vi "Send Write CPU View.vi"(7 "Message Priority (Normal)":T2=enum."Normal", 8 "error in (no error)":errorcluster, 10 "CPU View":T1 {"fwidth:" format="%#_6p"; "f0:" format="%#_6p"}, 11 "Message Enqueuer":refnum<class "Message Enqueuer.lvclass">) -> (0 "error out":errorcluster, 3 "Message Enqueuer out":refnum<class "Message Enqueuer.lvclass">)   [LabVIEW 2020, in "Simple UI.lvlib" / "Write CPU View Msg.lvclass"]
doc: "This VI sends the message to an actor."
uses:
  Write CPU View Msg.lvclass
  <vilib>/ActorFramework/Message Enqueuer/Message Enqueuer.lvclass
  <vilib>/ActorFramework/Message Enqueuer/Message Priority.ctl
  chart zoom.ctl
  C:/Program Files/National Instruments/LabVIEW 2026/vi.lib/ActorFramework/Message/Message.lvclass
  Write CPU View Msg.lvclass/Write CPU View Msg.ctl
  <vilib>/ActorFramework/Message Enqueuer/Message Enqueuer.lvclass/Message Enqueuer.ctl
  <vilib>/ActorFramework/Message Priority Queue/Priority Enqueue.vi
  Simple UI/Simple UI.lvclass
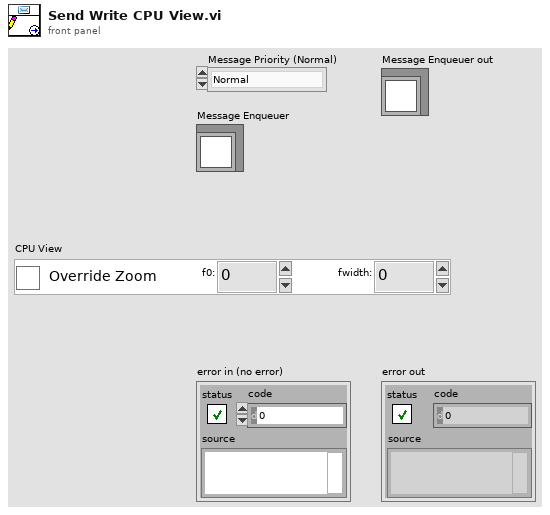
[diagram p1: front panel]
types:
  T1 = typedef "Simple UI.lvlib/Simple UI.lvclass/chart zoom.ctl" = cluster{"Override":bool, "f0: ":dbl, "fwidth: ":dbl}
  T2 = typedef "Actor Framework.lvlib/Message Enqueuer.lvclass/Message Priority.ctl" = enum16{"Low", "Normal", "High"}
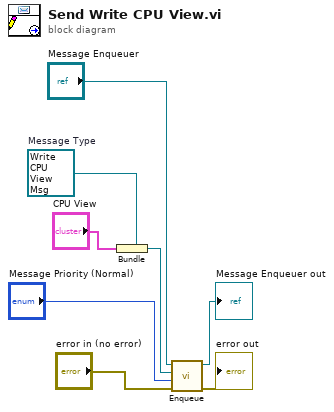
[diagram p0: block diagram]
diagram:
  w5 = refnum<class "Write CPU View Msg.lvclass"> refnum  # Message Type
  n1 = Bundle(cluster=w5, "CPU View") -> (w4:refnum<class "Write CPU View Msg.lvclass">)
  n2 = call <vilib>:"Enqueue.vi"("error in (no error)"="error in (no error)", "Message Priority (Normal)"="Message Priority (Normal)", "Message"=w4, "Message Enqueuer in"="Message Enqueuer") -> ("error out"=→"error out":errorcluster, "Message Enqueuer out"=→"Message Enqueuer out":refnum<class "Message Enqueuer.lvclass">)  [unwired: 6 in]
